vi "Verify CLI Output.vi"(4 "Execution time (s)":dbl=-1.0, 5 "Assert Only? (F)":bool, 6 "error code (1)":i32=1, 7 "Options":refnum<class "Options.lvclass">, 8 "error in":errorcluster, 9 "CLI Options":T1={"standard input"="", "working directory"=path "", "expected output size  (4096)"=4096, "Run Minimized (T)"=TRUE}, 10 "command line":string, 11 "Label":string) -> (0 "error out":errorcluster, 2 "Properties":refnum<class "Properties.Assert.lvclass">)   [LabVIEW 2020, in "Caraya.Extension.lvlib"]
doc: "Uses System Exec to execute command.\n\nCaptures:\nSTD out\nERR out\nReturn Code"
uses:
  Caraya.Extension.lvlib
  Approval Tests/Options/Options.lvclass
  <vilib>/addons/_JKI Toolkits/Caraya/classes/Properties.Assert/Properties.Assert.lvclass
  <vilib>/addons/_JKI Toolkits/Caraya/classes/Assert/Assert.lvclass
  <vilib>/addons/_JKI Toolkits/Caraya/classes/Assert/Assert True.vi
  Approval Tests/Approval Tests.lvlib
  Approval Tests/Verify CLI Options.ctl
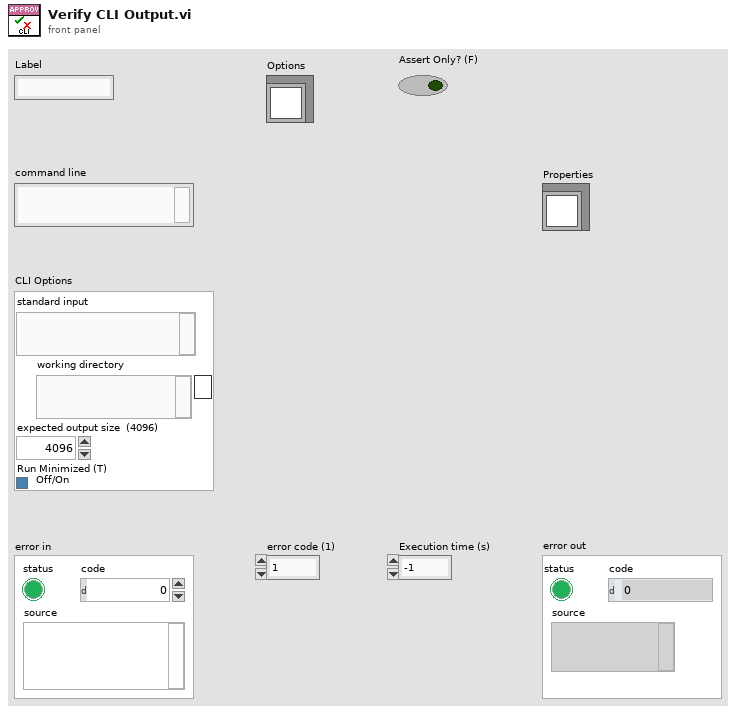
[diagram p1: front panel]
types:
  T1 = typedef "Approval Tests.lvlib/Verify CLI Options.ctl" = cluster{"standard input":string, "working directory":path, "expected output size  (4096)":u32, "Run Minimized (T)":bool}
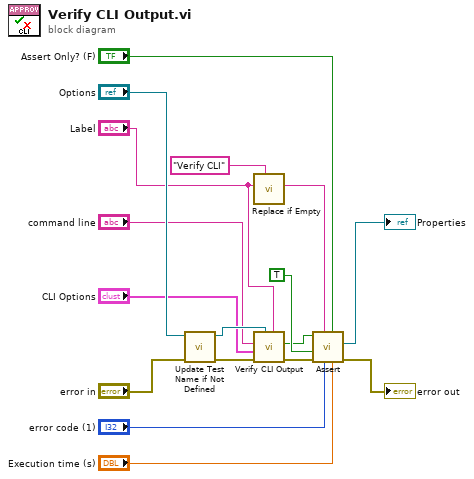
[diagram p0: block diagram]
diagram:
  n1 = call "Update Test Name if Not Defined.vi"("error in"="error in", "Options in"="Options") -> ("error out"=w14:errorcluster, "Options out"=w6:refnum<class "Options.lvclass">)  [unwired: 8 in]
  n2 = call "Replace if Empty.vi"("if empty"="Verify CLI" ("Label"), "Text in"="Label") -> ("Text out"=w1:string)  [unwired: 9 in]
  n3 = call "Verify CLI Output.vi"("Label"="Label", "Approval Tests.lvlib:Options.lvclass"=w6, "error in"=w14, "CLI Options"="CLI Options", "command line"="command line") -> ("error out"=w15:errorcluster, "Passed?"=w12:bool)  [unwired: 4 in, 1 out]
  n4 = call-poly <vilib>:"Assert.vi"("Execution time (s)"="Execution time (s)", "Assert Only? (F)"="Assert Only? (F)", "error code (1)"="error code (1)", "Label"=w1, "error in (no error)"=w15, "Register with caller test (F)"=TRUE, "True?"=w12) -> ("error out"=→"error out":errorcluster, "Properties"=→"Properties":refnum<class "Properties.Assert.lvclass">)  [unwired: 3 in]
